vi "Split_Layers.vi"(9 "#Active Layer":i32, 10 "Is Highlighted?":bool, 11 "Layer out":refnum<class "Layer.lvclass">[](array[class])) -> (1 "User Layers":refnum<class "Layer.lvclass">[](array[class]), 2 "Template":refnum<class "Layer.lvclass">, 3 "Icon Text":refnum<class "Layer.lvclass">)   [LabVIEW 2020]
uses:
  vi.lib/LabVIEW Icon API/lv_icon/Classes/Layer/Layer.lvclass
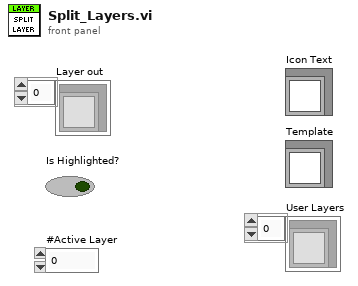
[diagram p1: front panel]
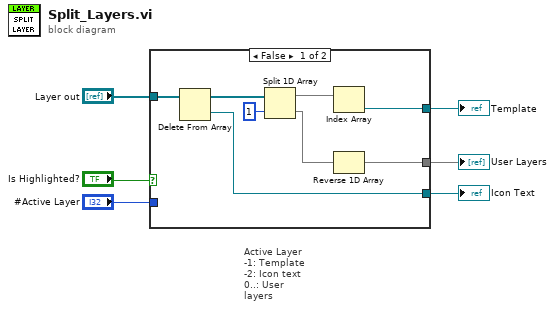
[diagram p0: block diagram]
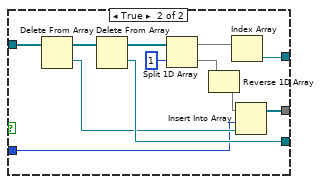
[diagram p2: hidden frame]
diagram:
  # "Active Layer\n-1: Template\n-2: Icon text\n0..: User layers"
  n1 = case shown="False" "Is Highlighted?" {
    tunnel: "Layer out" -> [w14 w26]
    tunnel: [w13 w21] -> w4
    tunnel: [w7 w18] -> w3
    tunnel: [w8 w20] -> w2
    tunnel: "#Active Layer" -> [_ w16]
    frame False {
      n2 = Delete From Array(array=w14) -> (deleted portion=w13:refnum<class "Layer.lvclass">, array with subset deleted=w12:refnum<class "Layer.lvclass">[])  [unwired: 2 in]
      n3 = Split 1D Array(array=w12, index=1) -> (first subarray=w9:refnum<class "Layer.lvclass">[], second subarray=w10:refnum<class "Layer.lvclass">[])
      n4 = Index Array(array=w9) -> (element=w8:refnum<class "Layer.lvclass">)  [unwired: 1 in]
      n5 = Reverse 1D Array(array=w10) -> (reversed array=w7:refnum<class "Layer.lvclass">[])
    }
    frame True {
      n6 = Delete From Array(array=w26) -> (deleted portion=w17:refnum<class "Layer.lvclass">, array with subset deleted=w25:refnum<class "Layer.lvclass">[])  [unwired: 2 in]
      n7 = Delete From Array(array=w25) -> (deleted portion=w21:refnum<class "Layer.lvclass">, array with subset deleted=w22:refnum<class "Layer.lvclass">[])  [unwired: 2 in]
      n8 = Split 1D Array(array=w22, index=1) -> (first subarray=w23:refnum<class "Layer.lvclass">[], second subarray=w19:refnum<class "Layer.lvclass">[])
      n9 = Reverse 1D Array(array=w19) -> (reversed array=w15:refnum<class "Layer.lvclass">[])
      n10 = Index Array(array=w23) -> (element=w20:refnum<class "Layer.lvclass">)  [unwired: 1 in]
      n11 = Insert Into Array(array=w15, index=w16, new element=w17) -> (w18:refnum<class "Layer.lvclass">[])
    }
  }
  "User Layers" <- w3
  "Template" <- w2
  "Icon Text" <- w4
